vi "Get Object Entry At.vi"(8 "error in":errorcluster, 10 "Index":i32, 11 "Obj Dict in":refnum<class "Object Dictionary.lvclass">) -> (0 "error out":errorcluster, 2 "Obj Entry":refnum<class "Object Entry.lvclass">, 3 "Obj Dict out":refnum<class "Object Dictionary.lvclass">)   [LabVIEW 2020, in "CANopen.lvlib" / "Object Dictionary.lvclass"]
doc: "Get Objects at specified index."
uses:
  Object Dictionary.lvclass
  Object Dictionary.lvclass/Object Dictionary.ctl
  Ordered-Dictionary/Ordered Object Dictionary/Source/Ordered Object Dictionary.lvclass
  Object Entry/Object Entry.lvclass
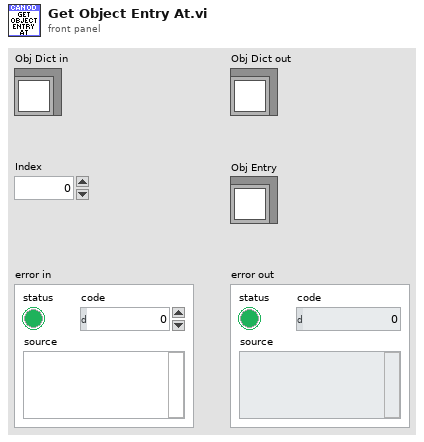
[diagram p1: front panel]
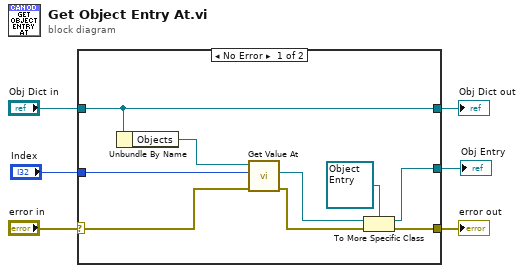
[diagram p0: block diagram]
diagram:
  n1 = case shown="No Error" "error in" {
    selector: "error in" -> [w12 w17]
    tunnel: [w10 w17] -> w3
    tunnel: [w15 w16] -> w5
    tunnel: "Obj Dict in" -> [w15 w16]
    tunnel: "Index" -> [w13 _]
    tunnel: [w7 _] -> w1
    frame No Error {
      n2 = Unbundle By Name(w15) -> ("Objects"=w14:refnum<class "Ordered Object Dictionary.lvclass">)
      n3 = call "Get Value At.vi"("error in"=w12, "Index"=w13, "Ordered Object Dictionary in"=w14) -> ("error out"=w11:errorcluster, "Value"=w8:refnum<class>)  [unwired: 6 in, 1 out]
      n4 = To More Specific Class(target class=refnum<class "Object Entry.lvclass"> refnum ("CANopen Object Dictionary.lvlib:Obj Entry"), reference=w8, error in=w11) -> (specific class reference=w7:refnum<class "Object Entry.lvclass">, error out=w10:errorcluster)
    }
    frame Error {
    }
  }
  "Obj Dict out" <- w5
  "error out" <- w3
  "Obj Entry" <- w1
